vi "Hall_analysis_Tsweep.vi"(4 "interpolation size":u16=2 min=2 step=1, 5 "max T":sgl=2.0 min=0 format="%.2f", 9 "Positive Tsweep data":string="2.000E+0\t-9.081E-1\t\n2.000E+0\t-9.082E-1\t\n2.000E+0\t-9.083E-1\t\n2.000E+0\t-9.081E-1\t\n2.000E+0\t-9.083E-1\t\n1.750E+0\t-9.075E-1\t\n1.750E+0\t-9.076E-1\t\n1.750E+0\t-9.073E-1\t\n1.750E+0\t-9.075E-1\t\n1.750E+0\t-9.075E-1\t\n1.500E+0\t-9.067E-1\t\n1.500E+0\t-9.068E-1\t\n1.500E+0\t-9.067E-1\t\n1.500E+0\t-9.067E-1\t\n1.500E+0\t-9.067E-1\t\n1.250E+0\t-9.057E-1\t\n1.250E+0\t-9.060E-1\t\n1.250E+0\t-9.059E-1\t\n1.250E+0\t-9.059E-1\t\n1.250E+0\t-9.057E-1\t\n1.000E+0\t-9.109E-1\t\n1.000E+0\t-9.109E-1\t\n1.000E+0\t-9.109E-1\t\n1.000E+0\t-9.108E-1\t\n1.000E+0\t-9.109E-1\t\n7.500E-1\t-9.041E-1\t\n7.500E-1\t-9.042E-1\t\n7.500E-1\t-9.042E-1\t\n7.500E-1\t-9.042E-1\t\n7.500E-1\t-9.042E-1\t\n5.000E-1\t-9.032E-1\t\n5.000E-1\t-9.031E-1\t\n2.000E+0\t-9.086E-1\t\n1.890E+0\t-9.080E-1\t\n1.780E+0\t-9.078E-1\t\n1.670E+0\t-9.074E-1\t\n1.560E+0\t-9.070E-1\t\n1.450E+0\t-9.068E-1\t\n1.340E+0\t-9.121E-1\t\n1.230E+0\t-9.058E-1\t\n1.120E+0\t-9.054E-1\t\n1.010E+0\t-9.111E-1\t\n9.000E-1\t-9.048E-1\t\n7.900E-1\t-9.044E-1\t\n6.800E-1\t-9.038E-1\t\n6.300E-1\t-9.037E-1\t\n5.800E-1\t-9.037E-1\t\n5.300E-1\t-9.033E-1\t\n4.800E-1\t-9.034E-1\t\n4.300E-1\t-9.029E-1\t\n3.800E-1\t-9.029E-1\t\n3.300E-1\t-9.043E-1\t\n2.800E-1\t-9.059E-1\t\n2.300E-1\t-9.135E-1\t\n1.800E-1\t-9.091E-1\t\n1.300E-1\t-9.108E-1\t\n8.000E-2\t-9.123E-1\t\n0.000E+0\t-9.211E-1\t") -> (1 "y(x)":cluster{"all rows":dbl[], "smoothed":dbl[]}[](graph)=[{"all rows"=[0.0, 0.08, 0.13, 0.18, 0.23, 0.28, 0.33, 0.38, 0.43, 0.48, 0.5, 0.5, 0.53, 0.58, 0.63, 0.68, 0.75, 0.75, 0.75, 0.75, 0.75, 0.79, 0.9, 1.0, 1.0, 1.0, 1.0, 1.0, 1.01, 1.12, 1.23, 1.25, 1.25, 1.25, 1.25, 1.25, 1.34, 1.45, 1.5, 1.5, 1.5, 1.5, 1.5, 1.56, 1.67, 1.75, 1.75, 1.75, 1.75, 1.75, 1.78, 1.89, 2.0, 2.0, 2.0, 2.0, 2.0, 2.0], "smoothed"=[-0.9211, -0.9123, -0.9108, -0.9091, -0.9135, -0.9059, -0.9043, -0.9029, -0.9029, -0.9034, -0.9032, -0.9031, -0.9033, -0.9037, -0.9037, -0.9038, -0.9041, -0.9042, -0.9042, -0.9042, -0.9042, -0.9044, -0.9048, -0.9109, -0.9109, -0.9109, -0.9108, -0.9109, -0.9111, -0.9054, -0.9058, -0.9057, -0.906, -0.9059, -0.9059, -0.9057, -0.9121, -0.9068, -0.9067, -0.9068, -0.9067, -0.9067, -0.9067, -0.907, -0.9074, -0.9075, -0.9076, -0.9073, -0.9075, -0.9075, -0.9078, -0.908, -0.9081, -0.9082, -0.9083, -0.9081, -0.9083, -0.9086]}, {"all rows"=[-0.11, -0.22, -0.33, -0.44, -0.55, -0.66, -0.77, -0.88, -0.99, -1.1, -1.21, -1.32, -1.43, -1.54, -1.65, -1.76], "smoothed"=[-0.9188, -0.9289, -0.9264, -0.9297, -0.9303, -0.9307, -0.9309, -0.9314, -0.9378, -0.9319, -0.9324, -0.9329, -0.9393, -0.9335, -0.934, -0.9343]}, {"all rows"=[0.0, 0.08, 0.13, 0.18, 0.23, 0.28, 0.33, 0.38, 0.43, 0.48, 0.5, 0.5, 0.53, 0.58, 0.63, 0.68, 0.75, 0.75, 0.75, 0.75, 0.75, 0.79, 0.9, 1.0, 1.0, 1.0, 1.0, 1.0, 1.01, 1.12, 1.23, 1.25, 1.25, 1.25, 1.25, 1.25, 1.34, 1.45, 1.5, 1.5, 1.5, 1.5, 1.5, 1.56, 1.67, 1.75, 1.75, 1.75, 1.75, 1.75, 1.78, 1.89, 2.0, 2.0, 2.0, 2.0, 2.0, 2.0], "smoothed"=[-0.9211, -0.9123, -0.9108, -0.9091, -0.9135, -0.9059, -0.9043, -0.9029, -0.9029, -0.9034, -0.9032, -0.9031, -0.9033, -0.9037, -0.9037, -0.9038, -0.9041, -0.9042, -0.9042, -0.9042, -0.9042, -0.9044, -0.9048, -0.9109, -0.9109, -0.9109, -0.9108, -0.9109, -0.9111, -0.9054, -0.9058, -0.9057, -0.906, -0.9059, -0.9059, -0.9057, -0.9121, -0.9068, -0.9067, -0.9068, -0.9067, -0.9067, -0.9067, -0.907, -0.9074, -0.9075, -0.9076, -0.9073, -0.9075, -0.9075, -0.9078, -0.908, -0.9081, -0.9082, -0.9083, -0.9081, -0.9083, -0.9086]}, {"all rows"=[-0.11, -0.22, -0.33, -0.44, -0.55, -0.66, -0.77, -0.88, -0.99, -1.1, -1.21, -1.32, -1.43, -1.54, -1.65, -1.76], "smoothed"=[-0.9188, -0.9289, -0.9264, -0.9297, -0.9303, -0.9307, -0.9309, -0.9314, -0.9378, -0.9319, -0.9324, -0.9329, -0.9393, -0.9335, -0.934, -0.9343]}], 3 "Result graph":cluster{dbl[], "Best Linear Fit":dbl[]}[](graph))   [LabVIEW 2025]
uses:
  <vilib>/Utility/file.llb/Read Delimited Spreadsheet (DBL).vi
  <vilib>/gmath/NI_Gmath.lvlib
panel:
  in  "method":i32(ring)=1 items=["nearest", "linear", "spline", "cubic Hermite", "Lagrange"]
  out "array w/ subset deleted 2":dbl[][](array[numeric])
  in  "min T":sgl=2.0 min=0 format="%.2f"
  out "negative data":dbl[][](array[numeric])=[[0.0, 0.08, 0.13, 0.18, 0.23, 0.28, 0.33, 0.38, 0.43, 0.48, 0.5, 0.5, 0.53, 0.58, 0.63, 0.68, 0.75, 0.75, 0.75, 0.75, 0.75, 0.79, 0.9, 1.0, 1.0, 1.0, 1.0, 1.0, 1.01, 1.12, 1.23, 1.25, 1.25, 1.25, 1.25, 1.25, 1.34, 1.45, 1.5, 1.5, 1.5, 1.5, 1.5, 1.56, 1.67, 1.75, 1.75, 1.75, 1.75, 1.75, 1.78, 1.89, 2.0, 2.0, 2.0, 2.0, 2.0, 2.0], [-0.9211, -0.9123, -0.9108, -0.9091, -0.9135, -0.9059, -0.9043, -0.9029, -0.9029, -0.9034, -0.9032, -0.9031, -0.9033, -0.9037, -0.9037, -0.9038, -0.9041, -0.9042, -0.9042, -0.9042, -0.9042, -0.9044, -0.9048, -0.9109, -0.9109, -0.9109, -0.9108, -0.9109, -0.9111, -0.9054, -0.9058, -0.9057, -0.906, -0.9059, -0.9059, -0.9057, -0.9121, -0.9068, -0.9067, -0.9068, -0.9067, -0.9067, -0.9067, -0.907, -0.9074, -0.9075, -0.9076, -0.9073, -0.9075, -0.9075, -0.9078, -0.908, -0.9081, -0.9082, -0.9083, -0.9081, -0.9083, -0.9086]]
  in  "Negative Tsweep data":string="2.000E+0\t-9.081E-1\t\n2.000E+0\t-9.082E-1\t\n2.000E+0\t-9.083E-1\t\n2.000E+0\t-9.081E-1\t\n2.000E+0\t-9.083E-1\t\n1.750E+0\t-9.075E-1\t\n1.750E+0\t-9.076E-1\t\n1.750E+0\t-9.073E-1\t\n1.750E+0\t-9.075E-1\t\n1.750E+0\t-9.075E-1\t\n1.500E+0\t-9.067E-1\t\n1.500E+0\t-9.068E-1\t\n1.500E+0\t-9.067E-1\t\n1.500E+0\t-9.067E-1\t\n1.500E+0\t-9.067E-1\t\n1.250E+0\t-9.057E-1\t\n1.250E+0\t-9.060E-1\t\n1.250E+0\t-9.059E-1\t\n1.250E+0\t-9.059E-1\t\n1.250E+0\t-9.057E-1\t\n1.000E+0\t-9.109E-1\t\n1.000E+0\t-9.109E-1\t\n1.000E+0\t-9.109E-1\t\n1.000E+0\t-9.108E-1\t\n1.000E+0\t-9.109E-1\t\n7.500E-1\t-9.041E-1\t\n7.500E-1\t-9.042E-1\t\n7.500E-1\t-9.042E-1\t\n7.500E-1\t-9.042E-1\t\n7.500E-1\t-9.042E-1\t\n5.000E-1\t-9.032E-1\t\n5.000E-1\t-9.031E-1\t\n2.000E+0\t-9.086E-1\t\n1.890E+0\t-9.080E-1\t\n1.780E+0\t-9.078E-1\t\n1.670E+0\t-9.074E-1\t\n1.560E+0\t-9.070E-1\t\n1.450E+0\t-9.068E-1\t\n1.340E+0\t-9.121E-1\t\n1.230E+0\t-9.058E-1\t\n1.120E+0\t-9.054E-1\t\n1.010E+0\t-9.111E-1\t\n9.000E-1\t-9.048E-1\t\n7.900E-1\t-9.044E-1\t\n6.800E-1\t-9.038E-1\t\n6.300E-1\t-9.037E-1\t\n5.800E-1\t-9.037E-1\t\n5.300E-1\t-9.033E-1\t\n4.800E-1\t-9.034E-1\t\n4.300E-1\t-9.029E-1\t\n3.800E-1\t-9.029E-1\t\n3.300E-1\t-9.043E-1\t\n2.800E-1\t-9.059E-1\t\n2.300E-1\t-9.135E-1\t\n1.800E-1\t-9.091E-1\t\n1.300E-1\t-9.108E-1\t\n8.000E-2\t-9.123E-1\t\n0.000E+0\t-9.211E-1\t"
  out "positive data":dbl[][](array[numeric])=[[0.0, 0.08, 0.13, 0.18, 0.23, 0.28, 0.33, 0.38, 0.43, 0.48, 0.5, 0.5, 0.53, 0.58, 0.63, 0.68, 0.75, 0.75, 0.75, 0.75, 0.75, 0.79, 0.9, 1.0, 1.0, 1.0, 1.0, 1.0, 1.01, 1.12, 1.23, 1.25, 1.25, 1.25, 1.25, 1.25, 1.34, 1.45, 1.5, 1.5, 1.5, 1.5, 1.5, 1.56, 1.67, 1.75, 1.75, 1.75, 1.75, 1.75, 1.78, 1.89, 2.0, 2.0, 2.0, 2.0, 2.0, 2.0], [-0.9211, -0.9123, -0.9108, -0.9091, -0.9135, -0.9059, -0.9043, -0.9029, -0.9029, -0.9034, -0.9032, -0.9031, -0.9033, -0.9037, -0.9037, -0.9038, -0.9041, -0.9042, -0.9042, -0.9042, -0.9042, -0.9044, -0.9048, -0.9109, -0.9109, -0.9109, -0.9108, -0.9109, -0.9111, -0.9054, -0.9058, -0.9057, -0.906, -0.9059, -0.9059, -0.9057, -0.9121, -0.9068, -0.9067, -0.9068, -0.9067, -0.9067, -0.9067, -0.907, -0.9074, -0.9075, -0.9076, -0.9073, -0.9075, -0.9075, -0.9078, -0.908, -0.9081, -0.9082, -0.9083, -0.9081, -0.9083, -0.9086]]
  in  "Negative sweep data file":path
  in  "Positive sweep data file":path=path "C:/work/data/PPMS/FeGaTe312_TC_THE_10K3"
  in  "Reload data file":bool
  in  "Data analyis method":T1(ring)
  in  "iteration Number":i32=2
  in  "smooth factor":i32=121
  in  "smooth":bool
  out "Tint PositiveInt NegativeInt Hall":string="-1.76000E+0\t-9.34300E-1\t0.00000E+0\t-1.15000E-3\r\n-1.65000E+0\t-9.34000E-1\t1.00000E-1\t3.55000E-3\r\n-1.54000E+0\t-9.33500E-1\t2.00000E-1\t8.10182E-3\r\n-1.43000E+0\t-9.39300E-1\t3.00000E-1\t1.09109E-2\r\n-1.32000E+0\t-9.32900E-1\t4.00000E-1\t1.28000E-2\r\n-1.21000E+0\t-9.32400E-1\t5.00000E-1\t1.34136E-2\r\n-1.10000E+0\t-9.31900E-1\t6.00000E-1\t1.33909E-2\r\n-9.90000E-1\t-9.37800E-1\t7.00000E-1\t1.34435E-2\r\n-8.80000E-1\t-9.31400E-1\t8.00000E-1\t1.33000E-2\r\n-7.70000E-1\t-9.30900E-1\t9.00000E-1\t1.38818E-2\r\n-6.60000E-1\t-9.30700E-1\t1.00000E+0\t1.31818E-2\r\n-5.50000E-1\t-9.30300E-1\t1.10000E+0\t1.27318E-2\r\n-4.40000E-1\t-9.29700E-1\t1.20000E+0\t1.33318E-2\r\n-3.30000E-1\t-9.26400E-1\t1.30000E+0\t1.17768E-2\r\n-2.20000E-1\t-9.28900E-1\t1.40000E+0\t1.41727E-2\r\n-1.10000E-1\t-9.18800E-1\t1.50000E+0\t1.44545E-2\r\n0.00000E+0\t-9.21100E-1\t1.60000E+0\t1.33136E-2\r\n8.00000E-2\t-9.12300E-1\t1.70000E+0\t1.33494E-2\r\n1.30000E-1\t-9.10800E-1\t1.80000E+0\t1.32318E-2\r\n1.80000E-1\t-9.09100E-1\t1.90000E+0\t1.31455E-2\r\n2.30000E-1\t-9.13500E-1\t2.00000E+0\t1.31000E-2\r\n2.80000E-1\t-9.05900E-1\t0.00000E+0\t0.00000E+0\r\n3.30000E-1\t-9.04300E-1\t0.00000E+0\t0.00000E+0\r\n3.80000E-1\t-9.02900E-1\t0.00000E+0\t0.00000E+0\r\n4.30000E-1\t-9.02900E-1\t0.00000E+0\t0.00000E+0\r\n4.80000E-1\t-9.03400E-1\t0.00000E+0\t0.00000E+0\r\n5.00000E-1\t-9.03200E-1\t0.00000E+0\t0.00000E+0\r\n5.00000E-1\t-9.03100E-1\t0.00000E+0\t0.00000E+0\r\n5.30000E-1\t-9.03300E-1\t0.00000E+0\t0.00000E+0\r\n5.80000E-1\t-9.03700E-1\t0.00000E+0\t0.00000E+0\r\n6.30000E-1\t-9.03700E-1\t0.00000E+0\t0.00000E+0\r\n6.80000E-1\t-9.03800E-1\t0.00000E+0\t0.00000E+0\r\n7.50000E-1\t-9.04100E-1\t0.00000E+0\t0.00000E+0\r\n7.50000E-1\t-9.04200E-1\t0.00000E+0\t0.00000E+0\r\n7.50000E-1\t-9.04200E-1\t0.00000E+0\t0.00000E+0\r\n7.50000E-1\t-9.04200E-1\t0.00000E+0\t0.00000E+0\r\n7.50000E-1\t-9.04200E-1\t0.00000E+0\t0.00000E+0\r\n7.90000E-1\t-9.04400E-1\t0.00000E+0\t0.00000E+0\r\n9.00000E-1\t-9.04800E-1\t0.00000E+0\t0.00000E+0\r\n1.00000E+0\t-9.10900E-1\t0.00000E+0\t0.00000E+0\r\n1.00000E+0\t-9.10900E-1\t0.00000E+0\t0.00000E+0\r\n1.00000E+0\t-9.10900E-1\t0.00000E+0\t0.00000E+0\r\n1.00000E+0\t-9.10800E-1\t0.00000E+0\t0.00000E+0\r\n1.00000E+0\t-9.10900E-1\t0.00000E+0\t0.00000E+0\r\n1.01000E+0\t-9.11100E-1\t0.00000E+0\t0.00000E+0\r\n1.12000E+0\t-9.05400E-1\t0.00000E+0\t0.00000E+0\r\n1.23000E+0\t-9.05800E-1\t0.00000E+0\t0.00000E+0\r\n1.25000E+0\t-9.05700E-1\t0.00000E+0\t0.00000E+0\r\n1.25000E+0\t-9.06000E-1\t0.00000E+0\t0.00000E+0\r\n1.25000E+0\t-9.05900E-1\t0.00000E+0\t0.00000E+0\r\n1.25000E+0\t-9.05900E-1\t0.00000E+0\t0.00000E+0\r\n1.25000E+0\t-9.05700E-1\t0.00000E+0\t0.00000E+0\r\n1.34000E+0\t-9.12100E-1\t0.00000E+0\t0.00000E+0\r\n1.45000E+0\t-9.06800E-1\t0.00000E+0\t0.00000E+0\r\n1.50000E+0\t-9.06700E-1\t0.00000E+0\t0.00000E+0\r\n1.50000E+0\t-9.06800E-1\t0.00000E+0\t0.00000E+0\r\n1.50000E+0\t-9.06700E-1\t0.00000E+0\t0.00000E+0\r\n1.50000E+0\t-9.06700E-1\t0.00000E+0\t0.00000E+0\r\n1.50000E+0\t-9.06700E-1\t0.00000E+0\t0.00000E+0\r\n1.56000E+0\t-9.07000E-1\t0.00000E+0\t0.00000E+0\r\n1.67000E+0\t-9.07400E-1\t0.00000E+0\t0.00000E+0\r\n1.75000E+0\t-9.07500E-1\t0.00000E+0\t0.00000E+0\r\n1.75000E+0\t-9.07600E-1\t0.00000E+0\t0.00000E+0\r\n1.75000E+0\t-9.07300E-1\t0.00000E+0\t0.00000E+0\r\n1.75000E+0\t-9.07500E-1\t0.00000E+0\t0.00000E+0\r\n1.75000E+0\t-9.07500E-1\t0.00000E+0\t0.00000E+0\r\n1.78000E+0\t-9.07800E-1\t0.00000E+0\t0.00000E+0\r\n1.89000E+0\t-9.08000E-1\t0.00000E+0\t0.00000E+0\r\n2.00000E+0\t-9.08100E-1\t0.00000E+0\t0.00000E+0\r\n2.00000E+0\t-9.08200E-1\t0.00000E+0\t0.00000E+0\r\n2.00000E+0\t-9.08300E-1\t0.00000E+0\t0.00000E+0\r\n2.00000E+0\t-9.08100E-1\t0.00000E+0\t0.00000E+0\r\n2.00000E+0\t-9.08300E-1\t0.00000E+0\t0.00000E+0\r\n2.00000E+0\t-9.08600E-1\t0.00000E+0\t0.00000E+0\r\n"
  in  "stop":bool
  in  "offset row":i32=1
  in  "data column":i32=2
  in  "Tcolumn":i32
  in  "(1) Data input method":T2(ring)
  # "linear fitting conditions"
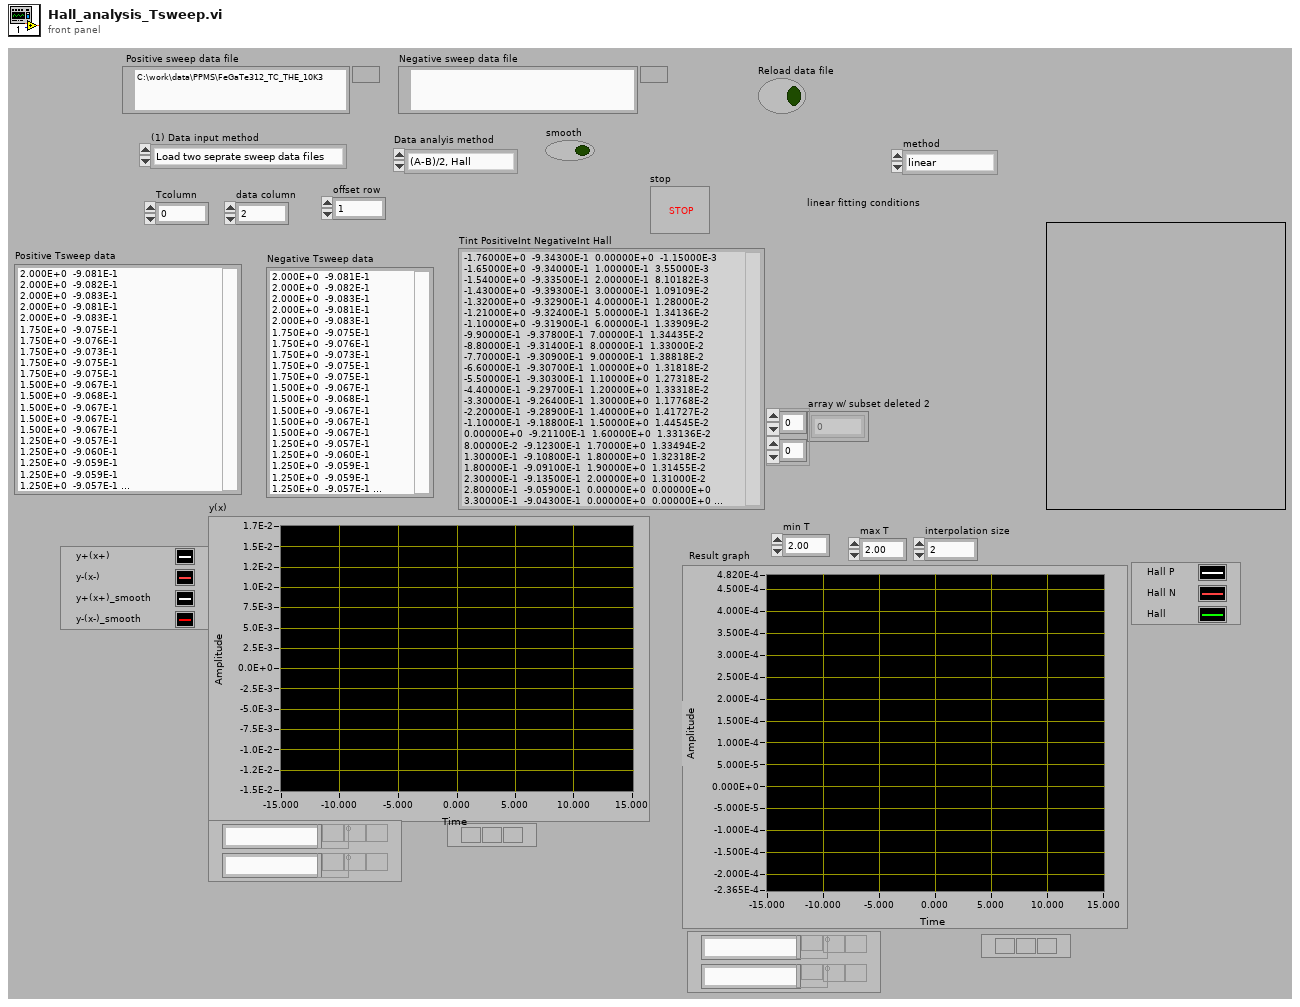
[diagram p1: front panel]
types:
  T1 = enum16{"(A-B)/2, Hall", "(A+B)/2, MR", "diagram defined"}
  T2 = enum16{"Load two seprate sweep data files", "Direct input (copy and paste)"}
  T3 = cluster{"negative data":dbl[], "negative data":dbl[]}
  T4 = cluster{" positive data":dbl[], "smoothed":dbl[]}
  T5 = cluster{" positive data":dbl[], " positive data":dbl[]}
  T6 = cluster{"negative data":dbl[], "smoothed":dbl[]}[]
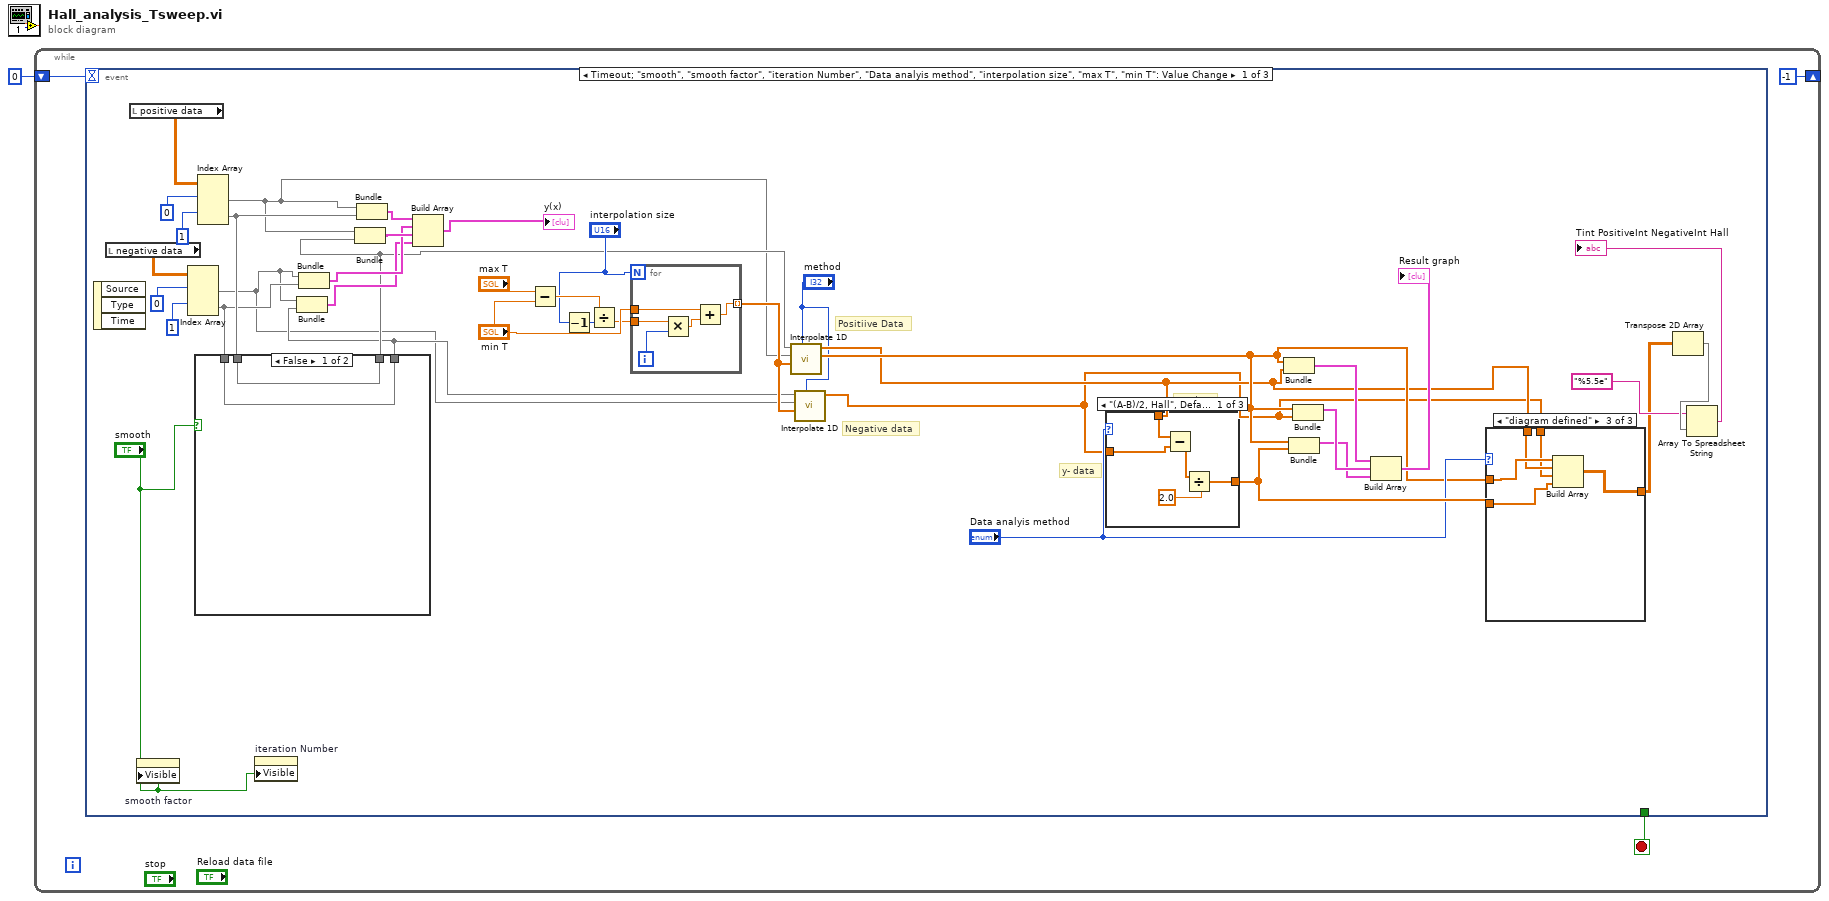
[diagram p0: block diagram]
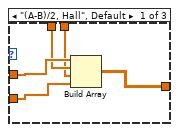
[diagram p2: hidden frame]
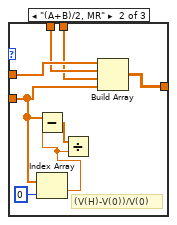
[diagram p3: hidden frame]
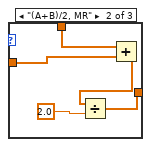
[diagram p4: hidden frame]
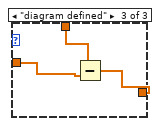
[diagram p5: hidden frame]
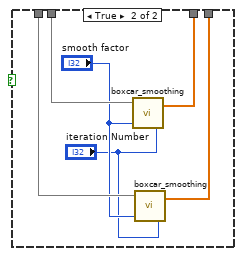
[diagram p6: hidden frame]
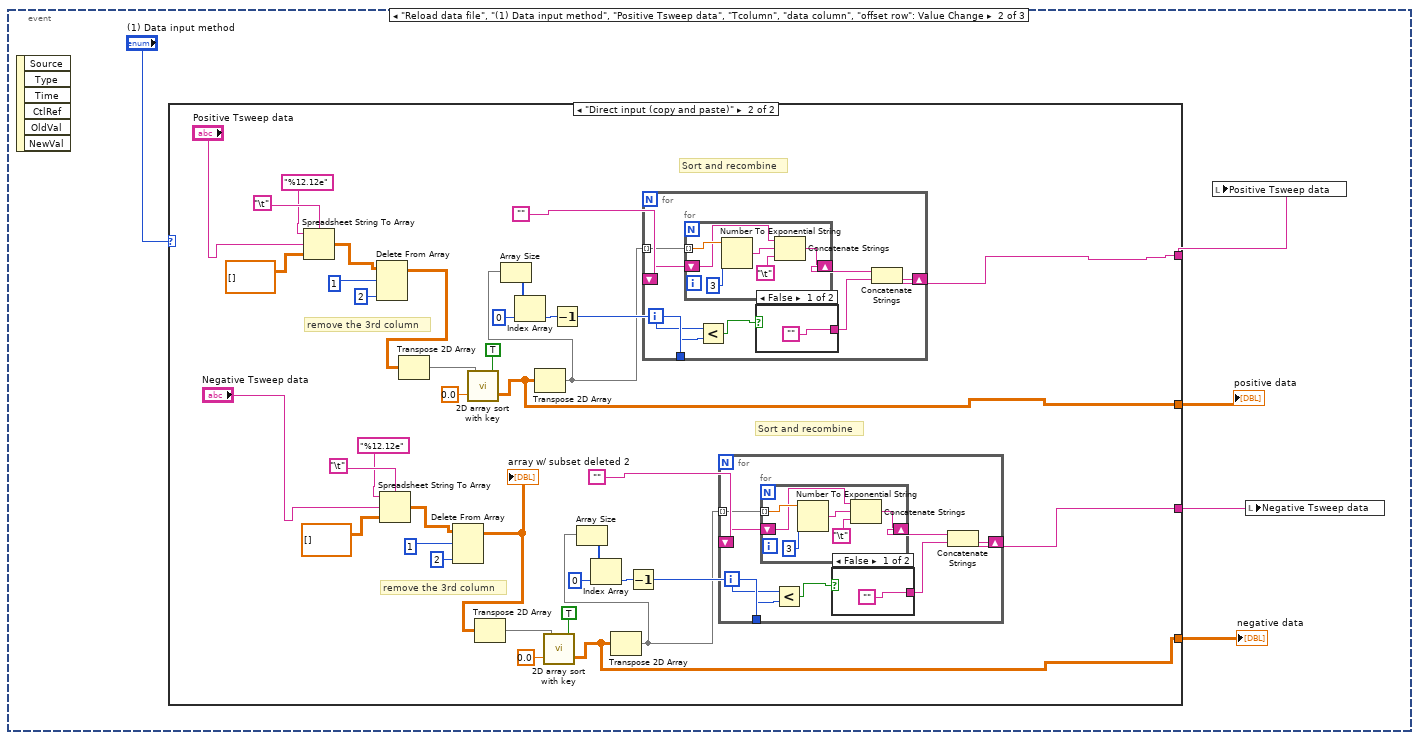
[diagram p7: hidden frame]
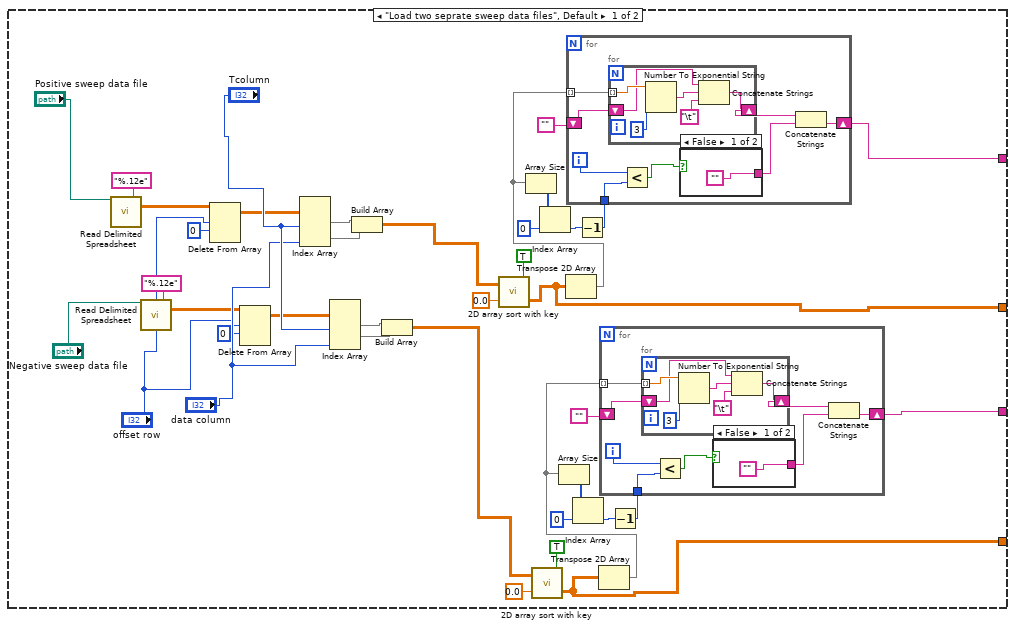
[diagram p8: hidden frame]
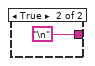
[diagram p9: hidden frame]
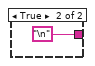
[diagram p10: hidden frame]
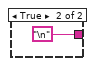
[diagram p11: hidden frame]
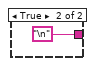
[diagram p12: hidden frame]
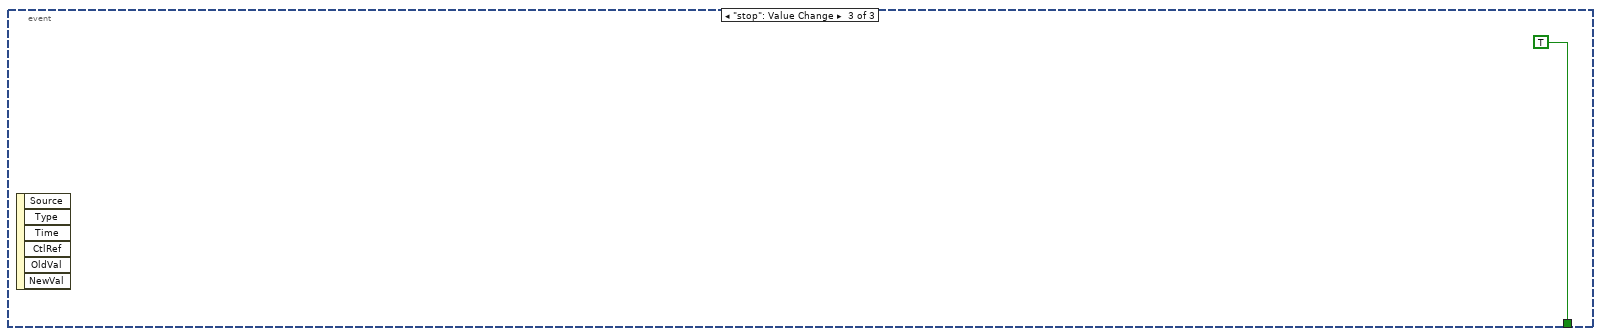
[diagram p13: hidden frame]
diagram:
  n1 = while {
    shift-right: [-1] -> _
    shift-left: 0 -> [w3]
    stop <- w4 stop-if-true
    n2 = event shown="[0] Timeout;  \"smooth\", \"smooth factor\", \"iteration Number\", \"Data analyis method\", \"interpolation size\", \"max T\", \"min T\": Value Change" {
      selector: _ -> [_ _ _]
      dyn-events: _ -> [_ _ _]
      timeout: w3 -> [_ _ _]
      tunnel: [_ _ TRUE] -> w4
      event Timeout; "smooth", "smooth factor", "iteration Number", "Data analyis method", "interpolation size", "max T", "min T": Value Change {
        # "y- data"
        # "Negative data"
        # "Positiive Data"
        # "y+ data"
        n3 = event-data() -> ()  [unwired: 1 in, 3 out]
        n4 = local read "negative data"() -> (w25:dbl[][])
        n5 = local read "positive data"() -> (w29:dbl[][])
        n6 = property on="smooth factor" class="DigNum (strict)"("Visible"="smooth") -> ()  [unwired: 2 in, 2 out]
        n7 = Index Array(array=w25, index (row) #1=0 ("disabled index (col)"), index (row) #2=1 ("index (col)")) -> (element #1=w5:dbl[], element #2=w9:dbl[])  [unwired: 2 in]
        n8 = Index Array(array=w29, index (row) #1=0 ("disabled index (col)"), index (row) #2=1 ("index (col)")) -> (element #1=w8:dbl[], element #2=w35:dbl[])  [unwired: 2 in]
        n9 = case shown="False" "smooth" {
          tunnel: w35 -> [w81 w87]
          tunnel: [w81 w86] -> w10
          tunnel: w9 -> [w80 w85]
          tunnel: [w80 w82] -> w6
          frame False {
          }
          frame True {
            n10 = call "boxcar_smoothing.vi"("iteration Number"="iteration Number", "smooth factor"="smooth factor", "raw data"=w87) -> ("smoothed"=w86:dbl[])  [unwired: 1 in]
            n11 = call "boxcar_smoothing.vi"("iteration Number"="iteration Number", "smooth factor"="smooth factor", "raw data"=w85) -> ("smoothed"=w82:dbl[])  [unwired: 1 in]
          }
        }
        n12 = property on="iteration Number" class="DigNum (strict)"("Visible"="smooth") -> ()  [unwired: 2 in, 2 out]
        n13 = Bundle("negative data"=w5, "smoothed"=w6) -> (w22:cluster{"negative data":dbl[], "smoothed":dbl[]})  [unwired: 1 out]
        n14 = Bundle("negative data"=w5, "negative data"=w9) -> (w23:T3)  [unwired: 1 out]
        n15 = Bundle("positive data"=w8, "smoothed"=w10) -> (w24:T4)  [unwired: 1 out]
        n16 = Bundle("positive data"=w8, "positive data"=w35) -> (w30:T5)  [unwired: 1 out]
        n17 = Build Array(w30, w23, w24, w22) -> (→"y(x)":T6)
        n18 = Subtract(x="max T", y="min T") -> (x-y=w20:sgl)
        n19 = Decrement(x="interpolation size") -> (x-1=w16:u16)
        n20 = Divide(x=w20, y=w16) -> (x/y=w17:sgl)
        n21 = for {
          N: "interpolation size" -> [_]
          tunnel: [w46] -> w15 mode=indexing
          tunnel: "min T" -> [w45]
          tunnel: w17 -> [w44]
          i -> [w48]
          n22 = Multiply(x=w44, y=w48) -> (x*y=w47:sgl)
          n23 = Add(x=w45, y=w47) -> (x+y=w46:sgl)
        }
        n24 = call <vilib>:"Interpolate 1D.vi"("method"="method", "xi"=w15, "X"=w8, "Y"=w10) -> ("xi used"=w14:dbl[], "yi"=w12:dbl[])  [unwired: 5 in, 1 out]
        n25 = call <vilib>:"Interpolate 1D.vi"("method"="method", "xi"=w15, "X"=w5, "Y"=w6) -> ("yi"=w11:dbl[])  [unwired: 5 in, 2 out]
        n26 = case shown="\"(A-B)/2, Hall\", Default" "Data analyis method" {
          tunnel: w12 -> [w71 w76 w79]
          tunnel: w11 -> [w68 w73 w78]
          tunnel: [w67 w72 w77] -> w31
          frame "(A-B)/2, Hall", Default {
            n27 = Subtract(x=w71, y=w68) -> (x-y=w69:dbl[])
            n28 = Divide(x=w69, y=2.0) -> (x/y=w67:dbl[])
          }
          frame "(A+B)/2, MR" {
            n29 = Add(x=w76, y=w73) -> (x+y=w74:dbl[])
            n30 = Divide(x=w74, y=2.0) -> (x/y=w72:dbl[])
          }
          frame "diagram defined" {
            n31 = Subtract(x=w79, y=w78) -> (x-y=w77:dbl[])
          }
        }
        n32 = Bundle("xi used"=w14, "yi"=w12) -> (w43:cluster{"xi used":dbl[], "yi":dbl[]})  [unwired: 1 out]
        n33 = Bundle("xi used"=w14, w31) -> (w41:cluster{"xi used":dbl[], dbl[]})  [unwired: 1 out]
        n34 = Bundle("xi used"=w14, "yi"=w11) -> (w42:cluster{"xi used":dbl[], "yi":dbl[]})  [unwired: 1 out]
        n35 = Build Array(w43, w42, w41) -> (→"Result graph":cluster{"xi used":dbl[], "yi":dbl[]}[])
        n36 = case shown="\"diagram defined\"" "Data analyis method" {
          tunnel: [w53 w57 w66] -> w13
          tunnel: w14 -> [w51 w56 w64]
          tunnel: w31 -> [w52 w60 w65]
          tunnel: w12 -> [w50 w55 w63]
          tunnel: w11 -> [w49 w54 w62]
          frame "(A-B)/2, Hall", Default {
            n37 = Build Array(w51, w50, w49, w52) -> (w53:dbl[][])
          }
          frame "(A+B)/2, MR" {
            # "(V(H)-V(0))/V(0)"
            n38 = Index Array(array=w60, index=0) -> (element=w58:dbl)
            n39 = Subtract(x=w60, y=w58) -> (x-y=w61:dbl[])
            n40 = Divide(x=w61, y=w58) -> ()  [unwired: 1 out]
            n41 = Build Array(w56, w55, w54, w60) -> (w57:dbl[][])
          }
          frame "diagram defined" {
            n42 = Build Array(w64, w63, w62, w65) -> (w66:dbl[][])
          }
        }
        n43 = Transpose 2D Array(2D array=w13) -> (transposed array=w39:dbl[][])
        n44 = Array To Spreadsheet String(array=w39, 3:"%5.5e" ("format string")) -> (spreadsheet string=→"Tint PositiveInt NegativeInt Hall":string)  [unwired: 1 out]
      }
      event "Reload data file", "(1) Data input method", "Positive Tsweep data", "Tcolumn", "data column", "offset row": Value Change {
        n45 = event-data() -> ()  [unwired: 1 in, 6 out]
        n46 = case shown="\"Direct input (copy and paste)\"" "(1) Data input method" {
          tunnel: [w120 w187] -> w92
          tunnel: [w118 w185] -> w91
          tunnel: [w108 w164] -> w90
          tunnel: [w107 w165] -> w89
          frame "Load two seprate sweep data files", Default {
            n47 = call-poly <vilib>:"Read Delimited Spreadsheet.vi"("file path (dialog if empty)"="Positive sweep data file", "format (%.3f)"="%.12e") -> ("all rows"=w102:dbl[][])  [unwired: 8 in, 5 out]
            n48 = call-poly <vilib>:"Read Delimited Spreadsheet.vi"("file path (dialog if empty)"="Negative sweep data file", "format (%.3f)"="%.12e") -> ("all rows"=w96:dbl[][])  [unwired: 8 in, 5 out]
            n49 = Delete From Array(array=w102, length="offset row", index (row)=0) -> (array with subset deleted=w101:dbl[][])  [unwired: 1 in, 1 out]
            n50 = Delete From Array(array=w96, length="offset row", index (row)=0) -> (array with subset deleted=w95:dbl[][])  [unwired: 1 in, 1 out]
            n51 = Index Array(array=w101, index (col) #1="Tcolumn", index (col) #2="data column") -> (element #1=w105:dbl[], element #2=w104:dbl[])  [unwired: 2 in]
            n52 = Index Array(array=w95, index (col) #1="Tcolumn", index (col) #2="data column") -> (element #1=w99:dbl[], element #2=w98:dbl[])  [unwired: 2 in]
            n53 = Build Array(w105, w104) -> (w93:dbl[][])
            n54 = Build Array(w99, w98) -> (w109:dbl[][])
            n55 = call "2D array sort with key.vi"("ascending"=TRUE, "key row"=0.0, "input"=w93) -> ("output"=w118:dbl[][])
            n56 = call "2D array sort with key.vi"("ascending"=TRUE, "key row"=0.0, "input"=w109) -> ("output"=w107:dbl[][])
            n57 = Transpose 2D Array(2D array=w118) -> (transposed array=w119:dbl[][])
            n58 = Array Size(array=w119) -> (size(s)=w126:i32[])
            n59 = Index Array(array=w126, index=0) -> (element=w124:i32)
            n60 = Decrement(x=w124) -> (x-1=w123:i32)
            n61 = for {
              tunnel: w119 -> [w155] mode=indexing
              shift-right: [w153] -> w120
              shift-left: "" -> [w152]
              tunnel: w123 -> [w148]
              i -> [w150]
              n62 = for {
                tunnel: w155 -> [w163] mode=indexing
                shift-right: [w159] -> w154
                shift-left: w152 -> [w160]
                n63 = Number To Exponential String(number=w163, precision (6)=i16 3) -> (E-format string=w161:string)  [unwired: 2 in]
                n64 = Concatenate Strings(w160, w161, "\t") -> (w159:string)
              }
              n65 = Less?(x=w150, y=w148) -> (x < y?=w149:bool)
              n66 = case shown="False" w149 {
                tunnel: ["" "\n"] -> w151
                frame False {
                }
                frame True {
                }
              }
              n67 = Concatenate Strings(w154, w151) -> (w153:string)
            }
            n68 = Transpose 2D Array(2D array=w107) -> (transposed array=w110:dbl[][])
            n69 = Array Size(array=w110) -> (size(s)=w116:i32[])
            n70 = Index Array(array=w116, index=0) -> (element=w114:i32)
            n71 = Decrement(x=w114) -> (x-1=w113:i32)
            n72 = for {
              tunnel: w110 -> [w139] mode=indexing
              shift-right: [w137] -> w108
              shift-left: "" -> [w136]
              tunnel: w113 -> [w132]
              i -> [w134]
              n73 = for {
                tunnel: w139 -> [w147] mode=indexing
                shift-right: [w143] -> w138
                shift-left: w136 -> [w144]
                n74 = Number To Exponential String(number=w147, precision (6)=i16 3) -> (E-format string=w145:string)  [unwired: 2 in]
                n75 = Concatenate Strings(w144, w145, "\t") -> (w143:string)
              }
              n76 = Less?(x=w134, y=w132) -> (x < y?=w133:bool)
              n77 = case shown="False" w133 {
                tunnel: ["" "\n"] -> w135
                frame False {
                }
                frame True {
                }
              }
              n78 = Concatenate Strings(w138, w135) -> (w137:string)
            }
          }
          frame "Direct input (copy and paste)" {
            # "Sort and recombine"
            # "remove the 3rd column"
            # "Sort and recombine"
            # "remove the 3rd column"
            n79 = Spreadsheet String To Array(delimiter (Tab)="\t", format string="%12.12e", spreadsheet string="Positive Tsweep data", array type (2D Dbl)=dbl[][] []) -> (array=w195:dbl[][])
            n80 = Delete From Array(array=w195, length=1, index (col)=2 ("disabled index (col)")) -> (array with subset deleted=w184:dbl[][])  [unwired: 1 in, 1 out]
            n81 = Spreadsheet String To Array(delimiter (Tab)="\t", format string="%12.12e", spreadsheet string="Negative Tsweep data", array type (2D Dbl)=dbl[][] []) -> (array=w177:dbl[][])
            n82 = Transpose 2D Array(2D array=w184) -> (transposed array=w183:dbl[][])
            n83 = Delete From Array(array=w177, length=1, index (col)=2 ("disabled index (col)")) -> (array with subset deleted=w168:dbl[][])  [unwired: 1 in, 1 out]
            "array w/ subset deleted 2" <- w168
            n84 = call "2D array sort with key.vi"("ascending"=TRUE, "key row"=0.0, "input"=w183) -> ("output"=w185:dbl[][])
            n85 = Transpose 2D Array(2D array=w168) -> (transposed array=w167:dbl[][])
            n86 = Transpose 2D Array(2D array=w185) -> (transposed array=w186:dbl[][])
            n87 = Array Size(array=w186) -> (size(s)=w193:i32[])
            n88 = Index Array(array=w193, index=0) -> (element=w191:i32)
            n89 = call "2D array sort with key.vi"("ascending"=TRUE, "key row"=0.0, "input"=w167) -> ("output"=w165:dbl[][])
            n90 = Decrement(x=w191) -> (x-1=w190:i32)
            n91 = Transpose 2D Array(2D array=w165) -> (transposed array=w169:dbl[][])
            n92 = Array Size(array=w169) -> (size(s)=w175:i32[])
            n93 = Index Array(array=w175, index=0) -> (element=w173:i32)
            n94 = Decrement(x=w173) -> (x-1=w172:i32)
            n95 = for {
              tunnel: w186 -> [w225] mode=indexing
              shift-right: [w223] -> w187
              shift-left: "" -> [w222]
              tunnel: w190 -> [w218]
              i -> [w220]
              n96 = for {
                tunnel: w225 -> [w233] mode=indexing
                shift-right: [w229] -> w224
                shift-left: w222 -> [w230]
                n97 = Number To Exponential String(number=w233, precision (6)=i16 3) -> (E-format string=w231:string)  [unwired: 2 in]
                n98 = Concatenate Strings(w230, w231, "\t") -> (w229:string)
              }
              n99 = Less?(x=w220, y=w218) -> (x < y?=w219:bool)
              n100 = case shown="False" w219 {
                tunnel: ["" "\n"] -> w221
                frame False {
                }
                frame True {
                }
              }
              n101 = Concatenate Strings(w224, w221) -> (w223:string)
            }
            n102 = for {
              tunnel: w169 -> [w209] mode=indexing
              shift-right: [w207] -> w164
              shift-left: "" -> [w206]
              tunnel: w172 -> [w202]
              i -> [w204]
              n103 = for {
                tunnel: w209 -> [w217] mode=indexing
                shift-right: [w213] -> w208
                shift-left: w206 -> [w214]
                n104 = Number To Exponential String(number=w217, precision (6)=i16 3) -> (E-format string=w215:string)  [unwired: 2 in]
                n105 = Concatenate Strings(w214, w215, "\t") -> (w213:string)
              }
              n106 = Less?(x=w204, y=w202) -> (x < y?=w203:bool)
              n107 = case shown="False" w203 {
                tunnel: ["" "\n"] -> w205
                frame False {
                }
                frame True {
                }
              }
              n108 = Concatenate Strings(w208, w205) -> (w207:string)
            }
          }
        }
        "positive data" <- w91
        "negative data" <- w89
        n109 = local write "Positive Tsweep data"(w92) -> ()
        n110 = local write "Negative Tsweep data"(w90) -> ()
      }
      event "stop": Value Change {
        n111 = event-data() -> ()  [unwired: 1 in, 6 out]
      }
    }
  }
